vi "DAQ Control.vi"(5 "Serial Configuration":T2={"Baud Rate"=9600, "Parity"=0, "Data Bits"=8, "Stop Bits"=10, "Flow Control"=0} {"Flow Control" items=["None", "XON/XOFF", "RTS/CTS", "XON/XOFF & RTS/CTS", "DTR/DSR", "XON/XOFF & DTR/DSR"]; "Stop Bits" items=["1.0"=10, "1.5"=15, "2.0"=20]; "Data Bits" items=["7"=7, "8"=8]; "Parity" items=["None", "Odd", "Even", "Mark", "Space"]; "Baud Rate" items=["300"=300, "600"=600, "1200"=1200, "2400"=2400, "4800"=4800, "9600"=9600, "19200"=19200]}, 6 "Throttle":dbl, 7 "Serial Port Configuration":T3={"baud rate (9600)"=115200, "data bits (8)"=8, "parity (0:none)"=enum."None"} {"data bits (8)" min=5 max=8 step=1}, 8 "?":bool, 9 "PSU VISA":refnum<visa-resource-name>, 10 "DAQ Device Name":tag="cDAQ1Mod1", 11 "Fuelflow VISA":refnum<visa-resource-name>) -> (1 "Power Supply Output":dbl[](array[numeric]), 2 "Power Output":cluster{"RPM":dbl, "Torque":dbl, "HP":dbl}, 3 "Fuelflow Output":T1, 4 "Mode":bool)   [LabVIEW 2014]
uses:
  <vilib>/Instr/_visa.llb/VISA Configure Serial Port (Instr).vi
  <vilib>/DAQmx/read.llb/DAQmx Read (Analog 1D DBL NChan 1Samp).vi
  <instrlib>/GPD-3303/GPD-3303.lvlib
panel:
  in  "Channel (1: Channel 1)":enum16{"Channel 1", "Channel 2"}(ring)=enum."Channel 2"
  out "Power supply Error Out":errorcluster
  out "Fuelflow Error Out":errorcluster
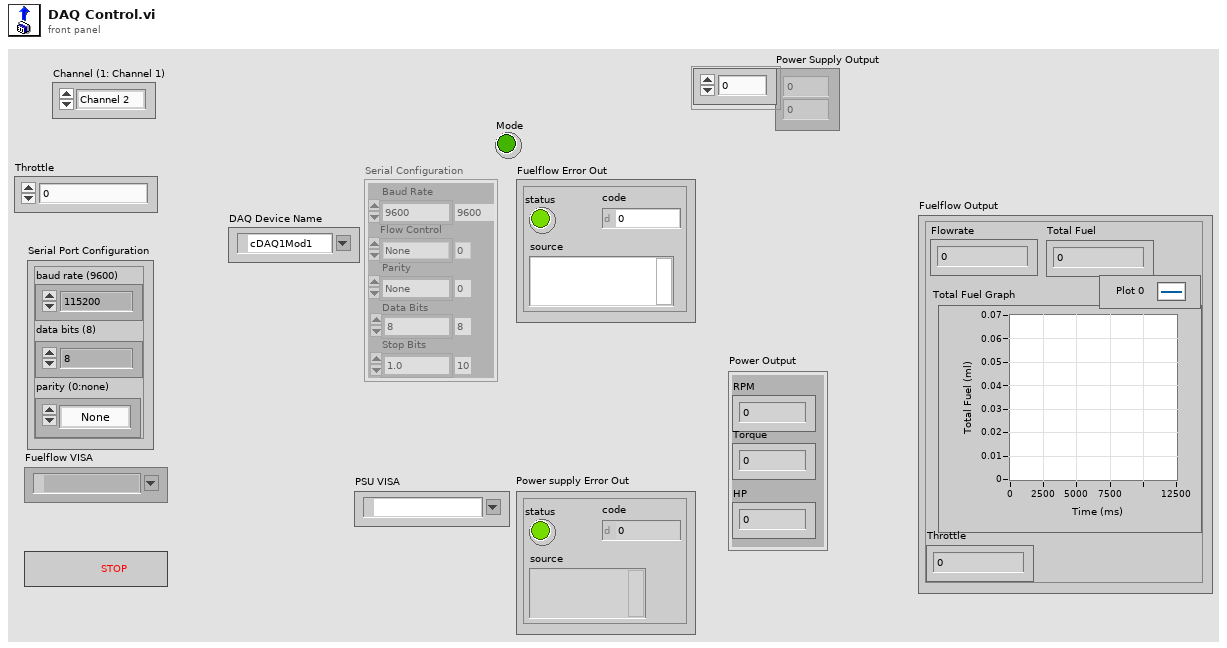
[diagram p1: front panel]
types:
  T1 = cluster{"Flowrate":dbl, "Total Fuel":dbl, "Total Fuel Graph":cluster{u32, dbl}[], "Throttle":dbl}
  T2 = cluster{"Baud Rate":u32, "Parity":u16, "Data Bits":u16, "Stop Bits":u16, "Flow Control":u16}
  T3 = cluster{"baud rate (9600)":u32, "data bits (8)":u16, "parity (0:none)":enum16{"None", "Odd", "Even", "Mark", "Space"}}
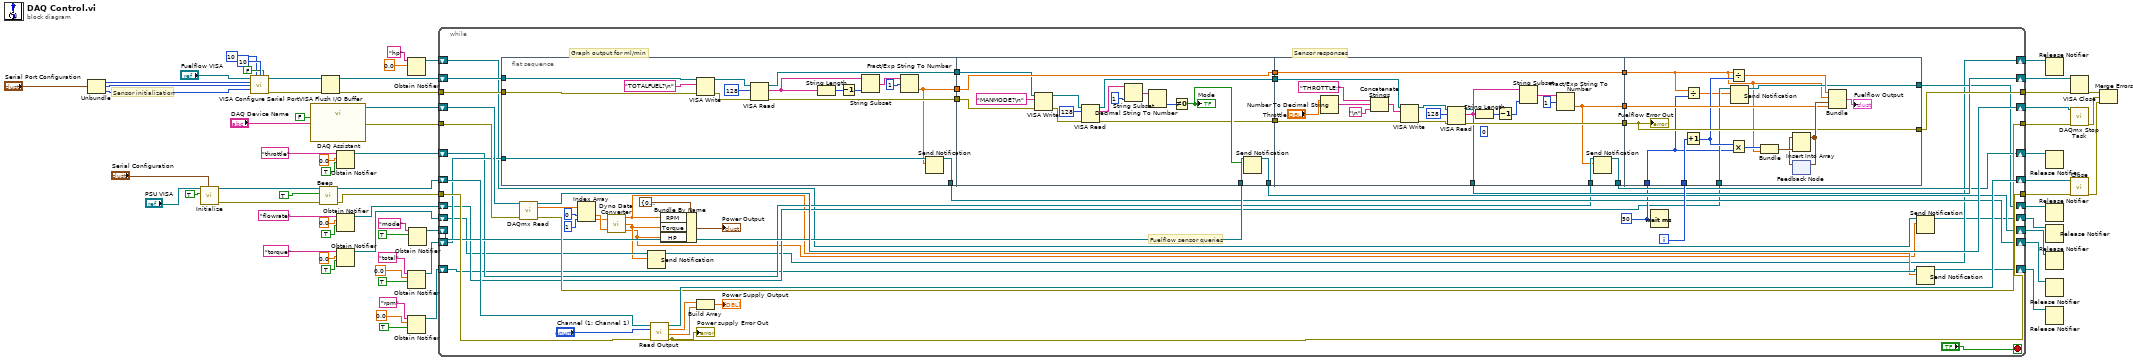
[diagram p0: block diagram]
diagram:
  # "Sensor initialization"
  n1 = Unbundle("Serial Port Configuration") -> ("baud rate (9600)"=w41:u32, "data bits (8)"=w40:u16, "parity (0:none)"=w39:enum16{"None", "Odd", "Even", "Mark", "Space"})
  n2 = call <instrlib>:"Initialize.vi"("Serial Configuration"="Serial Configuration", "ID Query (True)"=TRUE, "VISA resource name"="PSU VISA") -> ("error out"=w46:errorcluster, "VISA resource name out"=w47:refnum<visa-resource-name>)  [unwired: 7 in]
  n3 = call-poly "VISA Configure Serial Port"("VISA resource name"="Fuelflow VISA", "timeout (10sec)"=u32 10, "termination char\n(0xA = '\\n' = LF)"=u8 10 ("termination char\n(0xA = '\\n' = LF)"), "Enable Termination\nChar (T)"=FALSE ("Enable Termination\nChar (T)"), "baud rate (9600)"=w41, "data bits (8)"=w40, "parity (0:none)"=w39) -> ("VISA resource name out"=w42:refnum<visa-resource-name>, "error out"=w43:errorcluster)  [unwired: 7 in]
  n4 = call "DAQ Assistant"("stop (T)"=FALSE, "device name"="DAQ Device Name") -> ("task out"=w49:refnum<k21>, "error out"=w48:errorcluster)  [unwired: 15 in, 1 out]
  n5 = call <instrlib>:"Beep.vi"("error in (no error)"=w46, "Enable Beep (T: Enable)"=TRUE, "VISA resource name"=w47) -> ("error out"=w59:errorcluster, "VISA resource name out"=w58:refnum<visa-resource-name>)  [unwired: 7 in]
  n6 = VISA Flush I/O Buffer(VISA resource name=w42, error in (no error)=w43) -> (VISA resource name out=w38:refnum<visa-resource-name>, error out=w37:errorcluster)  [unwired: 1 in]
  n7 = Obtain Notifier(name (unnamed)="throttle", notification data type=0.0, create if not found? (T)=TRUE) -> (notifier out=w26:refnum<notifier>)  [unwired: 1 in, 2 out]
  n8 = Obtain Notifier(name (unnamed)="flowrate", notification data type=0.0, create if not found? (T)=TRUE) -> (notifier out=w22:refnum<notifier>)  [unwired: 1 in, 2 out]
  n9 = Obtain Notifier(name (unnamed)="torque", notification data type=0.0, create if not found? (T)=TRUE) -> (notifier out=w13:refnum<notifier>)  [unwired: 1 in, 2 out]
  n10 = Obtain Notifier(name (unnamed)="hp", notification data type=0.0) -> (notifier out=w14:refnum<notifier>)  [unwired: 2 in, 2 out]
  n11 = Obtain Notifier(name (unnamed)="total", notification data type=0.0, create if not found? (T)=TRUE) -> (notifier out=w27:refnum<notifier>)  [unwired: 1 in, 2 out]
  n12 = Obtain Notifier(name (unnamed)="rpm", notification data type=0.0, create if not found? (T)=TRUE) -> (notifier out=w15:refnum<notifier>)  [unwired: 1 in, 2 out]
  n13 = Obtain Notifier(name (unnamed)="mode", notification data type=TRUE) -> (notifier out=w34:refnum<notifier>)  [unwired: 2 in, 2 out]
  n14 = while {
    shift-right: [w97] -> w66
    shift-left: w38 -> [w98]
    shift-right: [w117] -> w64
    shift-left: w58 -> [w118]
    shift-right: [w111] -> w52
    shift-left: w49 -> [w112]
    shift-right: [w87] -> w4
    shift-left: w34 -> [w86]
    shift-right: [w82] -> w7
    shift-left: w27 -> [w81]
    shift-right: [w79] -> w8
    shift-left: w26 -> [w80]
    shift-right: [w76] -> w9
    shift-left: w22 -> [w77]
    shift-right: [w69] -> w6
    shift-left: w15 -> [w75]
    shift-right: [w68] -> w5
    shift-left: w14 -> [w73]
    shift-right: [w67] -> w10
    shift-left: w13 -> [w72]
    tunnel: w37 -> [w101]
    tunnel: [w99] -> w65
    tunnel: w48 -> [w113]
    tunnel: [w110] -> w51
    tunnel: w59 -> [w116]
    tunnel: [w115] -> w63
    i -> [w104]
    stop <- "?" stop-if-true
    w78 = u32 50 ("milliseconds to wait")
    # "Graph output for ml/min"
    # "Sensor responses"
    # "Fuelflow sensor queries"
    n15 = flat-sequence {
      tunnel: [w132] -> w93
      tunnel: [w131] -> w91
      tunnel: w98 -> [w133]
      tunnel: w101 -> [w134]
      tunnel: [w120] -> w89
      tunnel: w81 -> [w121]
      tunnel: [w119] -> w82
      tunnel: w93 -> [w149]
      tunnel: [w148] -> w92
      tunnel: w91 -> [w137]
      tunnel: [w135] -> w90
      tunnel: w89 -> [w150]
      tunnel: [w150] -> w88
      tunnel: w86 -> [w146]
      tunnel: [w144] -> w87
      tunnel: w92 -> [w171]
      tunnel: w90 -> [w170]
      tunnel: [w152] -> w103
      tunnel: [w169] -> w102
      tunnel: [w168] -> w100
      tunnel: [w167] -> w97
      tunnel: w88 -> [w169]
      tunnel: w80 -> [w154]
      tunnel: [w153] -> w79
      tunnel: w104 -> [w179]
      tunnel: w103 -> [w183]
      tunnel: w102 -> [w174]
      tunnel: w100 -> [w182]
      tunnel: [w182] -> w99
      tunnel: w78 -> [w173]
      tunnel: w77 -> [w176]
      tunnel: [w175] -> w76
      frame #0 {
        n16 = VISA Write(VISA resource name=w133, write buffer="TOTALFUEL?\n", error in (no error)=w134) -> (VISA resource name out=w127:refnum<visa-resource-name>, error out=w128:errorcluster)  [unwired: 1 out]
        n17 = VISA Read(VISA resource name=w127, byte count=128, error in (no error)=w128) -> (VISA resource name out=w132:refnum<visa-resource-name>, read buffer=w122:string, error out=w131:errorcluster)  [unwired: 1 out]
        n18 = String Length(string=w122) -> (length=w125:i32)
        n19 = Decrement(x=w125) -> (x-1=w124:i32)
        n20 = String Subset(string=w122, length (rest)=w124) -> (substring=w123:string)  [unwired: 1 in]
        n21 = Fract/Exp String To Number(string=w123, offset=1) -> (number=w120:dbl)  [unwired: 2 in, 1 out]
        n22 = Send Notification(notification=w120, notifier=w121) -> (notifier out=w119:refnum<notifier>)  [unwired: 1 in, 1 out]
      }
      frame #1 {
        n23 = VISA Write(VISA resource name=w149, write buffer="MANMODE?\n", error in (no error)=w137) -> (VISA resource name out=w143:refnum<visa-resource-name>, error out=w136:errorcluster)  [unwired: 1 out]
        n24 = VISA Read(VISA resource name=w143, byte count=u32 128, error in (no error)=w136) -> (VISA resource name out=w148:refnum<visa-resource-name>, read buffer=w140:string, error out=w135:errorcluster)  [unwired: 1 out]
        n25 = String Subset(string=w140, length (rest)=1 ("length (rest)")) -> (substring=w138:string)  [unwired: 1 in]
        n26 = Decimal String To Number(string=w138) -> (number=w147:i32)  [unwired: 2 in, 1 out]
        n27 = Not Equal To 0?(x=w147) -> (x != 0?=w145:bool)
        "Mode" <- w145
        n28 = Send Notification(notification=w145, notifier=w146) -> (notifier out=w144:refnum<notifier>)  [unwired: 1 in, 1 out]
      }
      frame #2 {
        (unwired) i16 0 ("width (-)")
        n29 = Number To Decimal String(number="Throttle") -> (decimal integer string=w162:string)  [unwired: 1 in]
        n30 = Concatenate Strings("THROTTLE:" ("string"), w162, "\n") -> (w160:string)
        n31 = VISA Write(VISA resource name=w171, write buffer=w160, error in (no error)=w170) -> (VISA resource name out=w165:refnum<visa-resource-name>, error out=w164:errorcluster)  [unwired: 1 out]
        n32 = VISA Read(VISA resource name=w165, byte count=128, error in (no error)=w164) -> (VISA resource name out=w167:refnum<visa-resource-name>, read buffer=w156:string, error out=w168:errorcluster)  [unwired: 1 out]
        n33 = String Length(string=w156) -> (length=w158:i32)
        n34 = Decrement(x=w158) -> (x-1=w157:i32)
        n35 = String Subset(string=w156, length (rest)=w157) -> (substring=w159:string)  [unwired: 1 in]
        n36 = Fract/Exp String To Number(string=w159, offset=1) -> (number=w152:dbl)  [unwired: 2 in, 1 out]
        n37 = Send Notification(notification=w152, notifier=w154) -> (notifier out=w153:refnum<notifier>)  [unwired: 1 in, 1 out]
      }
      frame #3 {
        n38 = Increment(x=w179) -> (x+1=w178:i32)
        n39 = Divide(x=w174, y=w173) -> (x/y=w172:dbl)
        n40 = Divide(x=w174, y=w178) -> (x/y=w181:dbl)
        n41 = Multiply(x=w178, y=w173) -> (x*y=w177:u32)
        n42 = Send Notification(notification=w172, notifier=w176) -> (notifier out=w175:refnum<notifier>)  [unwired: 1 in, 1 out]
        n43 = Bundle(w177, w174) -> (w186:cluster{u32, dbl})  [unwired: 1 in]
        n44 = feedback #1() -> (w185:cluster{u32, dbl}[])  [unwired: 1 in]
        n45 = Insert Into Array(array=w185, new element=w186) -> (w184:cluster{u32, dbl}[])  [unwired: 1 in]
        n46 = feedback-in #1(w184) -> ()
        n47 = Bundle(w181, w174, w184, w183) -> (→"Fuelflow Output":cluster{dbl, dbl, cluster{u32, dbl}[], dbl})  [unwired: 1 in]
        "Fuelflow Error Out" <- w182
      }
    }
    n48 = call-poly <vilib>:"DAQmx Read.vi"("task/channels in"=w112, "error in"=w113) -> ("task out"=w111:refnum<k21>, "data"=w109:dbl[], "error out"=w110:errorcluster)  [unwired: 11 in]
    n49 = Index Array(array=w109, index #1=0 ("index"), index #2=1 ("index")) -> (element #1=w106:dbl, element #2=w105:dbl)
    n50 = call "Dyno Data Converter.vi"("VShunt"=w105, "VGen"=w106) -> ("RPM"=w74:dbl, "Torque"=w71:dbl, "HP"=w70:dbl)
    n51 = Send Notification(notification=w71, notifier=w72) -> (notifier out=w68:refnum<notifier>)  [unwired: 1 in, 1 out]
    n52 = call <instrlib>:"Read Output.vi"("error in (no error)"=w116, "Channel (1: Channel 1)"="Channel (1: Channel 1)", "VISA resource name"=w118) -> ("error out"=w115:errorcluster, "Actual Current Level (A)"=w95:dbl, "Actual Voltage Level (V)"=w96:dbl, "VISA resource name out"=w117:refnum<visa-resource-name>)  [unwired: 5 in]
    "Power supply Error Out" <- w115
    n53 = Bundle By Name(cluster=cluster{"RPM":dbl, "Torque":dbl, "HP":dbl} {"RPM"=0.0, "Torque"=0.0, "HP"=0.0} ("Power Output"), "RPM"=w74, "Torque"=w71, "HP"=w70) -> (→"Power Output":cluster{"RPM":dbl, "Torque":dbl, "HP":dbl})
    n54 = Build Array(w96, w95) -> (→"Power Supply Output":dbl[])
    n55 = Wait (ms)(milliseconds to wait=w78) -> ()  [unwired: 1 out]
    n56 = Send Notification(notification=w70, notifier=w73) -> (notifier out=w67:refnum<notifier>)  [unwired: 1 in, 1 out]
    n57 = Send Notification(notification=w74, notifier=w75) -> (notifier out=w69:refnum<notifier>)  [unwired: 1 in, 1 out]
  }
  n58 = Release Notifier(notifier=w5) -> ()  [unwired: 2 in, 3 out]
  n59 = Release Notifier(notifier=w8) -> ()  [unwired: 2 in, 3 out]
  n60 = Release Notifier(notifier=w9) -> ()  [unwired: 2 in, 3 out]
  n61 = Release Notifier(notifier=w10) -> ()  [unwired: 2 in, 3 out]
  n62 = Release Notifier(notifier=w4) -> ()  [unwired: 2 in, 3 out]
  n63 = Release Notifier(notifier=w7) -> ()  [unwired: 2 in, 3 out]
  n64 = Release Notifier(notifier=w6) -> ()  [unwired: 2 in, 3 out]
  n65 = VISA Close(VISA resource name=w66, error in (no error)=w65) -> (error out=w62:errorcluster)
  n66 = call <vilib>:"DAQmx Stop Task.vi"("task/channels in"=w52, "error in"=w51) -> ("error out"=w53:errorcluster)  [unwired: 12 in, 1 out]
  n67 = call <instrlib>:"Close.vi"("error in (no error)"=w63, "VISA resource name"=w64) -> ("error out"=w54:errorcluster)  [unwired: 9 in]
  n68 = Merge Errors(w62, w53, w54) -> ()  [unwired: 1 out]
